vi "f_3_Qgtot_Vpl.vi"(0 "file path (IN)":path, 1 "Project #":string, 2 "Request #":string, 3 "TEST #":string, 5 "error in (no error)":errorcluster, 6 "VGE (-ve)":dbl, 8 "VGE (+ve)":dbl) -> (9 "Vpl":dbl, 11 "Di (A)":dbl, 13 "Dt (ns)":dbl, 14 "file path (OUT)":path, 15 "Qgtot - Delta Time (us)":dbl, 16 "Di/Dt (A/us)":dbl, 17 "DONE Qgtot & Vpl":bool, 18 "DONE Di/Dt ON":bool, 19 "error out":errorcluster)   [LabVIEW 2020]
uses:
  Global 1.vi
  <vilib>/measure/mamon.llb/Trigger Detection for 1 Channel.vi
  <vilib>/Analysis/NI_AALBase.lvlib
  <vilib>/measure/NI_MAPro.lvlib
panel:
  out "VGE (+ve) point":dbl
  out "Cursor c : Channel 2":dbl
  out "Find Major in Histogram":dbl
  out "Histogram":dynamicdata(graph)
  out "Focus graph":waveform(dbl)(graph)
  in  "Decision ?":bool
  out "Dt (us)":dbl
  out "VGE constant point in Median Filter":dbl
  out "VGE (-ve) point":dbl
  out "Cursor a : Channel 2":dbl
  out "Waveform Graph":waveform(dbl)[](graph)
  out "ON Region":waveform(dbl)[](graph) caption="Qgtot & Vpl"
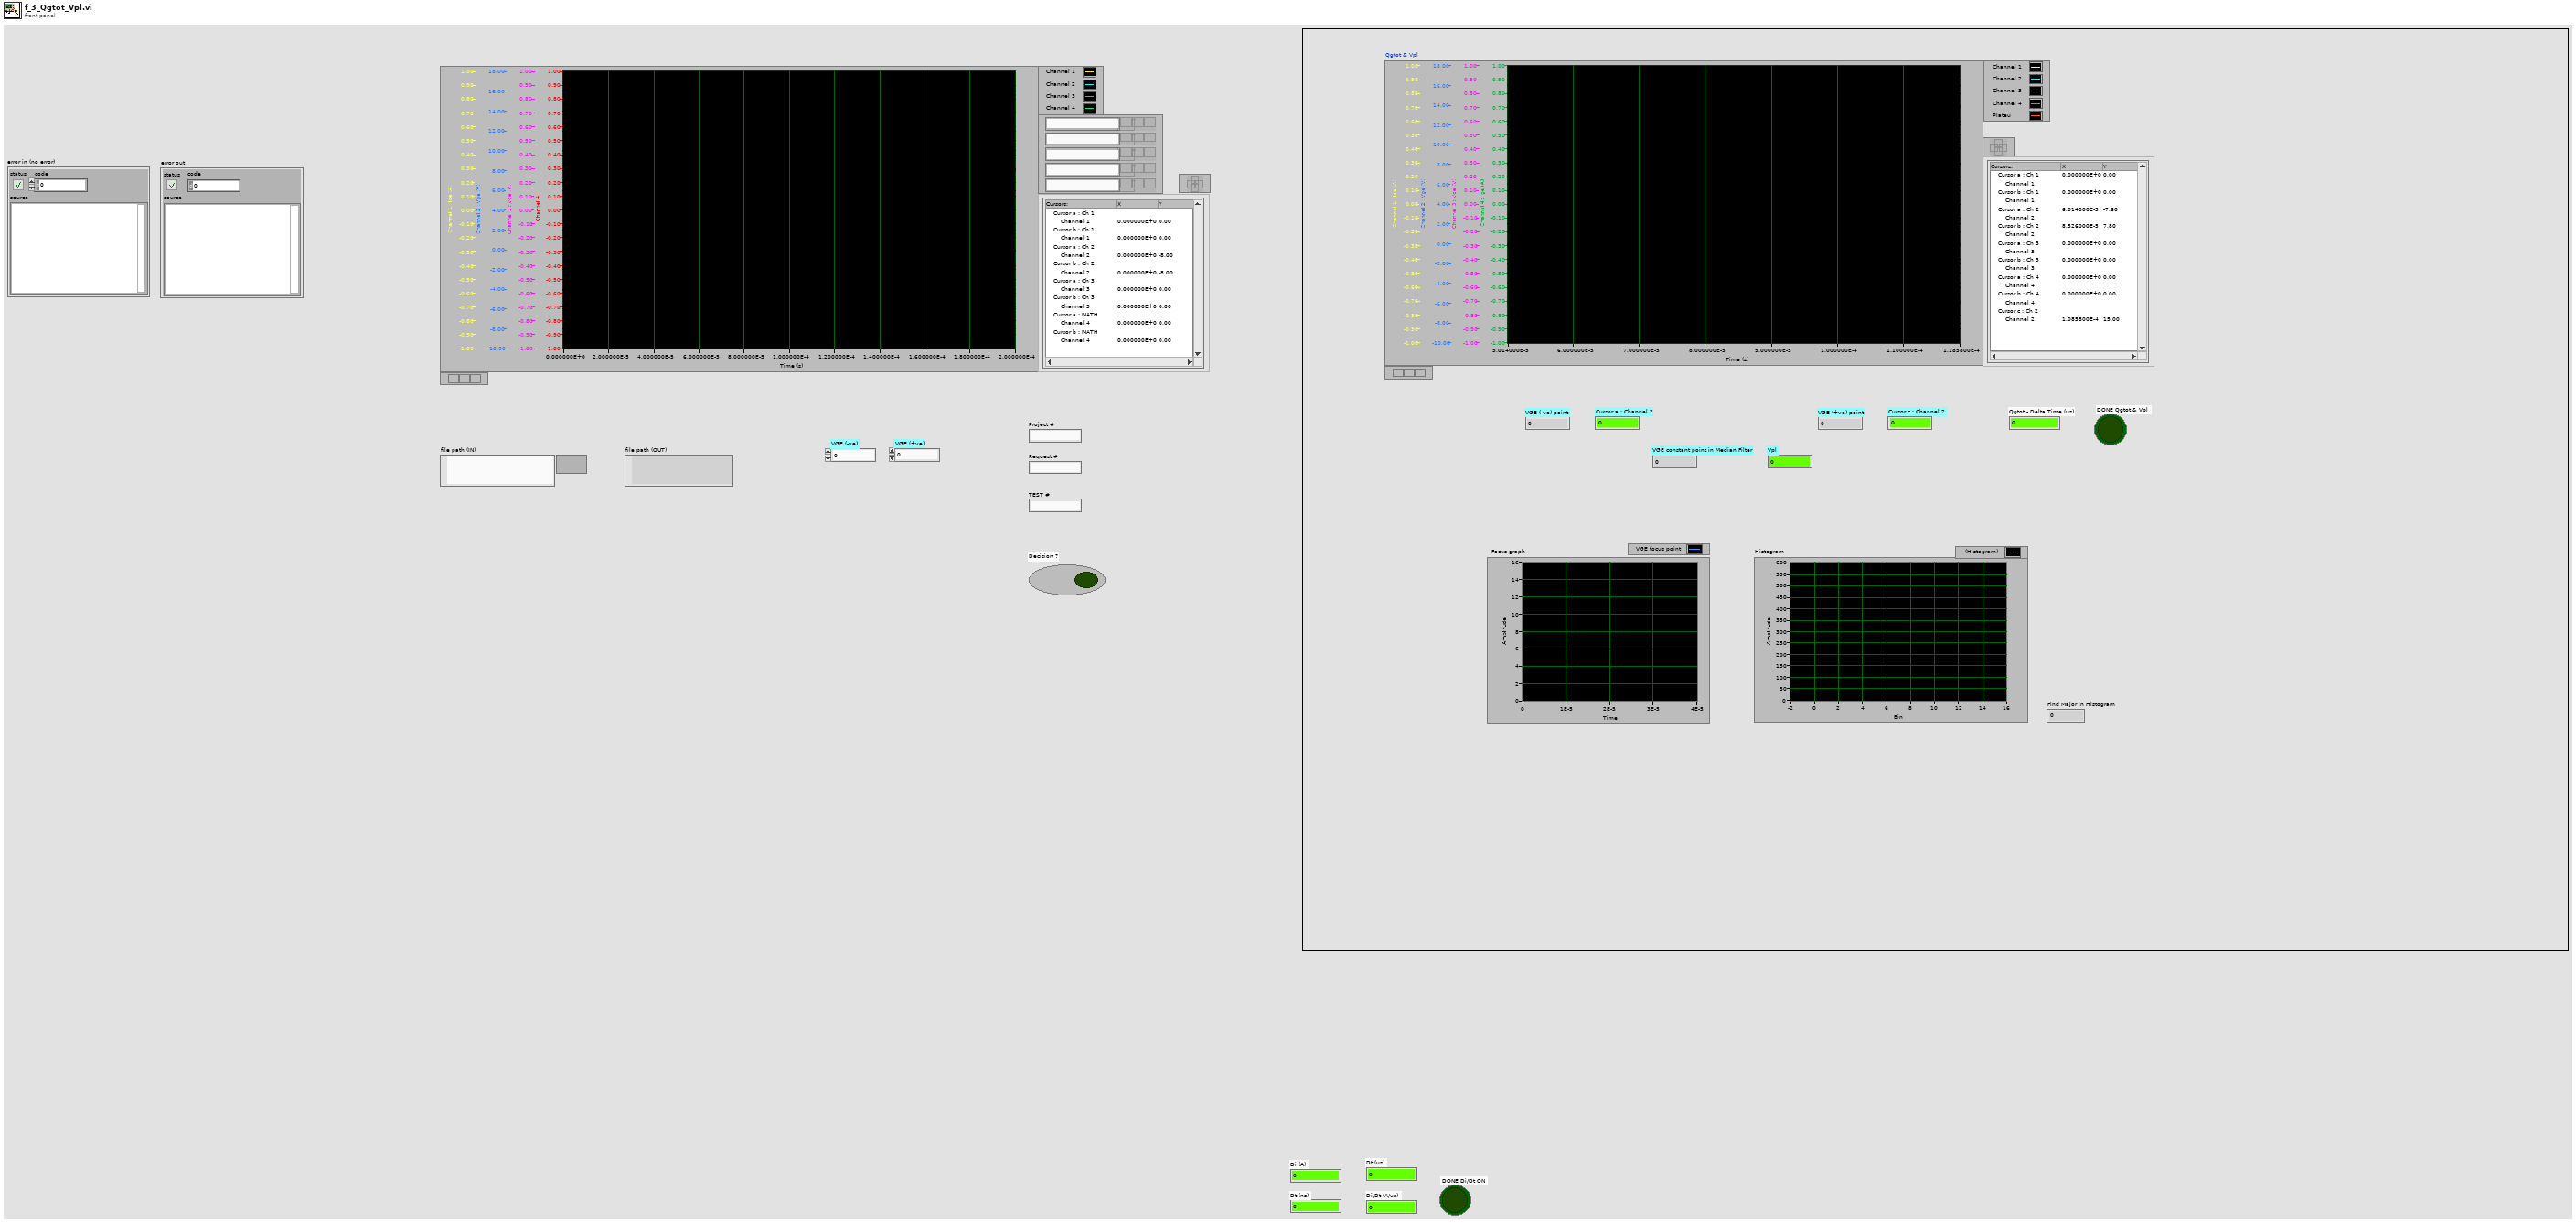
[diagram p1: front panel]
types:
  T1 = enum32{"Invalid", "Standard", "Closed", "Hidden", "Minimized", "Maximized"}
  T2 = typedef "imagedata.ctl" = cluster{"image type":i32, "image depth":i32, "image":u8[], "mask":u8[], "colors":u32[], "Rectangle":cluster{"left":i16, "top":i16, "right":i16, "bottom":i16}}
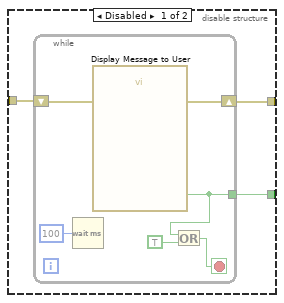
[diagram p2: hidden frame]
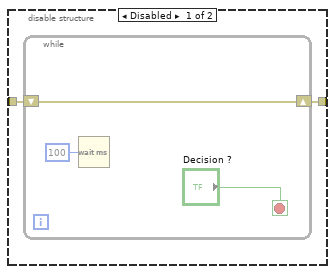
[diagram p10: hidden frame]
diagram:
  w5 = FALSE ("DONE Tdon")
  w1 = 0.0 ("Cursor a : Channel 1")
  w6 = errorcluster {"status"=FALSE, "code"=0, "source"=""} ("error out")
  w7 = waveform(dbl)[] [] ("Waveform Graph")
  n1 = local write "DONE Qgtot & Vpl"(w5) -> ()
  n2 = local write "VGE (-ve) point"(w1) -> ()
  n3 = local write "DONE Di/Dt ON"(w5) -> ()
  n4 = local write "Decision ?"(w5) -> ()
  n5 = local write "VGE constant point in Median Filter"(w1) -> ()
  n6 = local write "Di (A)"(w1) -> ()
  n7 = local write "Dt (ns)"(w1) -> ()
  n8 = local write "Dt (us)"(w1) -> ()
  n9 = local write "Di/Dt (A/us)"(w1) -> ()
  n10 = local write "VGE (+ve) point"(w1) -> ()
  n11 = local write "Cursor c : Channel 2"(w1) -> ()
  n12 = local write "Find Major in Histogram"(0.0 ("Time of Maximum")) -> ()
  n13 = local write "error out"(w6) -> ()
  n14 = local write "error in (no error)"(w6) -> ()
  n15 = local write "Cursor a : Channel 2"(w1) -> ()
  n16 = local write "Vpl"(w1) -> ()
  n17 = local write "Qgtot - Delta Time (us)"(w1) -> ()
  n18 = local write "Waveform Graph"(w7) -> ()
  n19 = local write "ON Region"(w7) -> ()
  n20 = local write "Histogram"(dynamicdata [] ("Histogram")) -> ()
  n21 = local write "Focus graph"(waveform(dbl) {"t0"=timestamp(0 s since 1904-01-01), "dt"=1.0, "Y"=[]} ("Focus graph")) -> ()
  n22 = flat-sequence {
    tunnel: ["file path (IN)"] -> w13
    tunnel: [w14] -> w12
    tunnel: [w23] -> w11
    tunnel: [w22] -> w10
    tunnel: w13 -> [w25]
    tunnel: w12 -> [w24]
    tunnel: [w314] -> w9
    tunnel: w11 -> [w313]
    tunnel: w10 -> [w312]
    tunnel: [w312] -> w8
    tunnel: w9 -> [w329]
    tunnel: w8 -> [w328]
    frame #0 {
      n23 = control-ref of="This VI"() -> (w19:refnum<vi>)
      n24 = invoke class="VI" method="FP.Open"(reference=w19, error in="error in (no error)", "Activate"=TRUE ("Activate?"), "State"=T1."Maximized") -> (error out=w20:errorcluster)  [unwired: 1 in, 4 out]
      n25 = property class="VI"(reference=w19, error in=w20, "Front Panel.Closeable"=TRUE ("Front Panel Window:Closeable")) -> (error out=w14:errorcluster)  [unwired: 1 out]
    }
    frame #1 {
      n26 = while {
        tunnel: w25 -> [w57]
        shift-right: [w52] -> w23
        shift-left: w24 -> [w56]
        tunnel: [w54] -> w22
        stop <- w51 stop-if-true
        n27 = flat-sequence {
          tunnel: [w86] -> w67
          tunnel: [w87] -> w66
          tunnel: w57 -> [w87]
          tunnel: w56 -> [w86]
          tunnel: w67 -> [w105]
          tunnel: w66 -> [w103]
          tunnel: [w102] -> w47
          tunnel: [w94] -> w46
          tunnel: [w88] -> w45
          tunnel: [w90] -> w44
          tunnel: [w91] -> w43
          tunnel: [w89] -> w42
          tunnel: [w92] -> w41
          tunnel: w47 -> [w145]
          tunnel: [w145] -> w40
          tunnel: w46 -> [w144]
          tunnel: [w144] -> w38
          tunnel: w45 -> [w136]
          tunnel: w44 -> [_]
          tunnel: w43 -> [w143]
          tunnel: w42 -> [w142]
          tunnel: [w142] -> w39
          tunnel: w41 -> [w141]
          tunnel: [w134] -> w37
          tunnel: [w157] -> w50
          tunnel: w40 -> [w215]
          tunnel: [w215] -> w49
          tunnel: w39 -> [w214]
          tunnel: [w214] -> w48
          tunnel: w38 -> [w171]
          tunnel: w37 -> [w164]
          tunnel: w50 -> [w228]
          tunnel: [w236] -> w36
          tunnel: w49 -> [w244]
          tunnel: [w244] -> w35
          tunnel: [w232] -> w33
          tunnel: [w229] -> w29
          tunnel: w48 -> [w216]
          tunnel: [w216] -> w26
          tunnel: w36 -> [w261]
          tunnel: w35 -> [w266]
          tunnel: [w266] -> w34
          tunnel: w33 -> [w265]
          tunnel: [w265] -> w32
          tunnel: [w249] -> w31
          tunnel: [w251] -> w30
          tunnel: w29 -> [w264]
          tunnel: [w264] -> w28
          tunnel: [w252] -> w27
          tunnel: w26 -> [w259]
          tunnel: [w269] -> w65
          tunnel: w34 -> [w274]
          tunnel: [w274] -> w64
          tunnel: w32 -> [w273]
          tunnel: [w273] -> w63
          tunnel: w31 -> [w272]
          tunnel: [w272] -> w62
          tunnel: w30 -> [w267]
          tunnel: [w267] -> w61
          tunnel: w28 -> [w271]
          tunnel: [w271] -> w60
          tunnel: w27 -> [w270]
          tunnel: w65 -> [w286]
          tunnel: w64 -> [w298]
          tunnel: [w298] -> w59
          tunnel: w63 -> [w293]
          tunnel: w62 -> [w294]
          tunnel: w61 -> [w292]
          tunnel: w60 -> [w291]
          tunnel: [w286] -> w58
          tunnel: w59 -> [w303]
          tunnel: w58 -> [w305]
          tunnel: [w304] -> w53
          tunnel: [w303] -> w54
          frame #0 {
            w83 = waveform(dbl)[] [] ("Waveform Graph")
            w79 = 0.0 ("Cursor a : Channel 1")
            w85 = FALSE ("DONE Tdon")
            n28 = local write "DONE Qgtot & Vpl"(w85) -> ()
            n29 = local write "Cursor a : Channel 2"(w79) -> ()
            n30 = local write "Di (A)"(w79) -> ()
            n31 = local write "Dt (ns)"(w79) -> ()
            n32 = local write "Dt (us)"(w79) -> ()
            n33 = local write "Di/Dt (A/us)"(w79) -> ()
            n34 = local write "DONE Di/Dt ON"(w85) -> ()
            n35 = local write "Decision ?"(w85) -> ()
            n36 = local write "Find Major in Histogram"(w79) -> ()
            n37 = local write "VGE constant point in Median Filter"(w79) -> ()
            n38 = local write "VGE (-ve) point"(w79) -> ()
            n39 = local write "VGE (+ve) point"(w79) -> ()
            n40 = local write "Cursor c : Channel 2"(w79) -> ()
            n41 = local write "Qgtot - Delta Time (us)"(w79) -> ()
            n42 = Wait (ms)(milliseconds to wait=u32 200) -> ()  [unwired: 1 out]
            n43 = local write "Vpl"(w79) -> ()
            n44 = Wait (ms)(milliseconds to wait=u32 200) -> ()  [unwired: 1 out]
            n45 = local write "Histogram"(dynamicdata [] ("Histogram")) -> ()
            n46 = local write "ON Region"(w83) -> ()
            n47 = local write "Waveform Graph"(w83) -> ()
            n48 = local write "Focus graph"(waveform(dbl) {"t0"=timestamp(0 s since 1904-01-01), "dt"=1.0, "Y"=[]} ("Focus graph")) -> ()
          }
          frame #1 {
            w94 = 0.0 ("number")
            # "Channel 2"
            # "Channel 4"
            # "t0"
            # "Channel 1"
            # "Channel 3"
            # "dt"
            # "Ch1"
            n49 = call "3_ReadDatatoWaveform.vi"("file path (IN)"=w103, "error in (no error)"=w105) -> ("Ch 1 Data"=w101:dbl[], "Ch 2 Data"=w96:dbl[], "file path (OUT)"=w102:path, "Waveform Graph"=→"Waveform Graph":waveform(dbl)[], "Ch 3 Data"=w100:dbl[], "Ch 4 Data"=w98:dbl[], "dt"=w91:dbl, "error out"=w104:errorcluster)  [unwired: 5 in, 1 out]
            n50 = To Time Stamp(1:w94) -> (0:w97:timestamp)
            n51 = disable-structure shown="Enabled" {
              disable-tunnel: w97 -> [w121 _]
              disable-tunnel: w91 -> [w120 _]
              disable-tunnel: w96 -> [w119 _]
              disable-tunnel: [w118 _] -> w90
              frame Enabled {
                # "Channel 2"
                n52 = Bundle By Name("Y"=w119, "dt"=w120, "t0"=w121) -> (w118:waveform(dbl))  [unwired: 1 in]
              }
              frame Disabled {
              }
            }
            n53 = disable-structure shown="Enabled" {
              disable-tunnel: w97 -> [w133 _]
              disable-tunnel: w91 -> [w132 _]
              disable-tunnel: w100 -> [w131 _]
              disable-tunnel: [w130 _] -> w106
              frame Enabled {
                # "Channel 3"
                n54 = Bundle By Name("Y"=w131, "dt"=w132, "t0"=w133) -> (w130:waveform(dbl))  [unwired: 1 in]
              }
              frame Disabled {
              }
            }
            n55 = disable-structure shown="Enabled" {
              disable-tunnel: w97 -> [w125 _]
              disable-tunnel: w91 -> [w124 _]
              disable-tunnel: w98 -> [w123 _]
              disable-tunnel: [w122 _] -> w93
              frame Enabled {
                # "Channel 4"
                n56 = Bundle By Name("Y"=w123, "dt"=w124, "t0"=w125) -> (w122:waveform(dbl))  [unwired: 1 in]
              }
              frame Disabled {
              }
            }
            n57 = disable-structure shown="Enabled" {
              disable-tunnel: w97 -> [w129 _]
              disable-tunnel: w91 -> [w128 _]
              disable-tunnel: w101 -> [w127 _]
              disable-tunnel: [w126 _] -> w107
              frame Enabled {
                # "Channel 1"
                n58 = Bundle By Name("Y"=w127, "dt"=w128, "t0"=w129) -> (w126:waveform(dbl))  [unwired: 1 in]
              }
              frame Disabled {
              }
            }
            n59 = property on="Waveform Graph" class="WFGraph (strict)"(error in=w104, "XScale.Offset"=w94) -> (error out=w88:errorcluster)  [unwired: 1 in, 1 out]
            n60 = disable-structure shown="Enabled" {
              disable-tunnel: w90 -> [w116 _]
              disable-tunnel: [w115 _] -> w89
              disable-tunnel: [w114 _] -> w92
              disable-tunnel: w91 -> [w113 _]
              frame Enabled {
                # "OG = 30"
                # "Median"
                n61 = global read "Global 1.vi" "Median Filter Rank"() -> (w112:i32)
                n62 = Unbundle By Name(w116) -> ("Y"=w117:dbl[])
                n63 = call <vilib>:"Median Filter.vi"("right rank"=w112, "left rank"=w112, "X"=w117) -> ("Filtered X"=w114:dbl[])  [unwired: 7 in, 1 out]
                n64 = Bundle By Name("Y"=w114, "dt"=w113) -> (w115:waveform(dbl))  [unwired: 1 in]
              }
              frame Disabled {
              }
            }
            n65 = Build Array(w107, w90, w106, w93, w89) -> (→"ON Region":waveform(dbl)[])
            n66 = Wait (ms)(milliseconds to wait=u32 200) -> ()  [unwired: 1 out]
            n67 = call <vilib>:"Beep.vi"("use system alert? (T)"=FALSE, "duration (msec)"=u32 200, "frequency (Hz)"=u32 2000) -> ()  [unwired: 9 in]
          }
          frame #2 {
            n68 = disable-structure shown="Enabled" {
              disable-tunnel: w143 -> [_ w151]
              disable-tunnel: w141 -> [_ w147]
              disable-tunnel: [_ w146] -> w139
              frame Disabled {
              }
              frame Enabled {
                # "Remains"
                # "Find (+ve)"
                # "Find 0"
                n69 = Search 1D Array(1D array=w147, element=0.0, start index (0)=0) -> (index of element=w152:i32)
                n70 = Split 1D Array(array=w147, index=w152) -> (second subarray=w155:dbl[])  [unwired: 1 out]
                n71 = Search 1D Array(1D array=w155, element="VGE (+ve)", start index (0)=0) -> (index of element=w154:i32)
                n72 = Split 1D Array(array=w155, index=w154) -> (first subarray=w156:dbl[])  [unwired: 1 out]
                n73 = Bundle By Name("Y"=w156, "dt"=w151) -> (w146:waveform(dbl))  [unwired: 1 in]
                "Focus graph" <- w146
              }
            }
            n74 = Wait (ms)(milliseconds to wait=u32 200) -> ()  [unwired: 1 out]
            n75 = call "Create Histogram"("error in (no error)"=w136, "Signal"=w139) -> ("error out"=w135:errorcluster, "Histogram"=w138:dynamicdata)  [unwired: 8 in]
            "Histogram" <- w138
            n76 = call "Statistics"("Signals"=w138, "error in (no error)"=w135) -> ("Time of Maximum"=→"Find Major in Histogram":dynamicdata, "error out"=w134:errorcluster)  [unwired: 24 in]
          }
          frame #3 {
            n77 = property on="ON Region" class="WFGraph (strict)"(error in=w164) -> (error out=w172:errorcluster, "Width"=w173:u32)  [unwired: 1 in, 1 out]
            n78 = property on="ON Region" class="WFGraph (strict)"(error in=w172, "Caption.Justify"=enum16{"Left", "Center", "Right"}."Left" ("Caption.Justification"), "Caption.Width"=w173, "Caption.FontBold"=TRUE ("Caption.Font:Bold"), "Caption.FontColor"=u32 16860 ("Caption.Font:Color"), "Caption.FontSize"=u32 24 ("Caption.Font:Size"), "Caption.Text"="Qgtot & Vpl") -> (error out=w174:errorcluster)  [unwired: 1 in, 1 out]
            n79 = Wait (ms)(milliseconds to wait=u32 200) -> ()  [unwired: 1 out]
            n80 = property on="ON Region" class="WFGraph (strict)"(error in=w174, "XScale.Offset"=w171) -> (error out=w165:errorcluster)  [unwired: 1 in, 1 out]
            n81 = property on="ON Region" class="WFGraph (strict)"(error in=w165, "Active Cursor"=u32 0, "Cursor.Cursor X"=0.0 ("Cursor.Cursor Position:Cursor X"), "Cursor.Cursor Y"=0.0 ("Cursor.Cursor Position:Cursor Y"), "Cursor.Visible"=FALSE) -> (error out=w207:errorcluster)  [unwired: 1 in, 1 out]
            n82 = property on="ON Region" class="WFGraph (strict)"(error in=w207, "Active Cursor"=u32 1, "Cursor.Cursor X"=0.0 ("Cursor.Cursor Position:Cursor X"), "Cursor.Cursor Y"=0.0 ("Cursor.Cursor Position:Cursor Y"), "Cursor.Visible"=FALSE) -> (error out=w208:errorcluster)  [unwired: 1 in, 1 out]
            n83 = property on="ON Region" class="WFGraph (strict)"(error in=w208, "Active Cursor"=u32 2, "Cursor.Cursor X"=0.0 ("Cursor.Cursor Position:Cursor X"), "Cursor.Cursor Y"=0.0 ("Cursor.Cursor Position:Cursor Y"), "Cursor.Visible"=FALSE) -> (error out=w209:errorcluster)  [unwired: 1 in, 1 out]
            n84 = property on="ON Region" class="WFGraph (strict)"(error in=w209, "Active Cursor"=u32 3, "Cursor.Cursor X"=0.0 ("Cursor.Cursor Position:Cursor X"), "Cursor.Cursor Y"=0.0 ("Cursor.Cursor Position:Cursor Y"), "Cursor.Visible"=FALSE) -> (error out=w210:errorcluster)  [unwired: 1 in, 1 out]
            n85 = property on="ON Region" class="WFGraph (strict)"(error in=w210, "Active Cursor"=u32 4, "Cursor.Cursor X"=0.0 ("Cursor.Cursor Position:Cursor X"), "Cursor.Cursor Y"=0.0 ("Cursor.Cursor Position:Cursor Y"), "Cursor.Visible"=FALSE) -> (error out=w211:errorcluster)  [unwired: 1 in, 1 out]
            n86 = property on="ON Region" class="WFGraph (strict)"(error in=w211, "Active Cursor"=u32 5, "Cursor.Cursor X"=0.0 ("Cursor.Cursor Position:Cursor X"), "Cursor.Cursor Y"=0.0 ("Cursor.Cursor Position:Cursor Y"), "Cursor.Visible"=FALSE) -> (error out=w212:errorcluster)  [unwired: 1 in, 1 out]
            n87 = property on="ON Region" class="WFGraph (strict)"(error in=w212, "Active Cursor"=u32 6, "Cursor.Cursor X"=0.0 ("Cursor.Cursor Position:Cursor X"), "Cursor.Cursor Y"=0.0 ("Cursor.Cursor Position:Cursor Y"), "Cursor.Visible"=FALSE) -> (error out=w213:errorcluster)  [unwired: 1 in, 1 out]
            n88 = property on="ON Region" class="WFGraph (strict)"(error in=w213, "Active Cursor"=u32 7, "Cursor.Cursor X"=0.0 ("Cursor.Cursor Position:Cursor X"), "Cursor.Cursor Y"=0.0 ("Cursor.Cursor Position:Cursor Y"), "Cursor.Visible"=FALSE) -> (error out=w158:errorcluster)  [unwired: 1 in, 1 out]
            n89 = property on="ON Region" class="WFGraph (strict)"(error in=w158, "Active Cursor"=u32 8, "Cursor.Cursor X"=0.0 ("Cursor.Cursor Position:Cursor X"), "Cursor.Cursor Y"=0.0 ("Cursor.Cursor Position:Cursor Y"), "Cursor.Visible"=FALSE) -> (error out=w157:errorcluster)  [unwired: 1 in, 1 out]
          }
          frame #4 {
            w225 = u16 1 items=["Falling Edge", "Rising Edge"] ("trigger slope")
            w226 = u16 1 items=["Index", "Time"] ("location mode")
            w230 = u16 1 items=["Falling Edge", "Rising Edge"] ("trigger slope")
            w231 = u16 1 items=["Index", "Time"] ("location mode")
            # "Cursor a : Channel 2"
            # "Cursor a : Channel 2"
            # "Cursor b : Channel 2"
            # "Cursor a : Channel 2"
            # "Cursor b : Channel 2"
            # "Cursor a : Channel 2"
            # "End Time 1st Cursor"
            # "End Time 2nd Cursor"
            # "1st PARAMETER : VGE (-ve)"
            # "Channel 2"
            # "2nd PARAMETER : VGE constant point"
            # "Channel 2"
            n90 = Add(x="VGE (-ve)", y=0.3) -> (x+y=w219:dbl)
            n91 = call-poly <vilib>:"Basic Level Trigger Detection.vi"("signal in"=w216, "level"=w219, "location mode"=w231, "error in (no error)"=w228, "trigger slope"=w230) -> ("trigger location"=w229:dbl, "error out"=w227:errorcluster)  [unwired: 8 in, 1 out]
            n92 = property on="ON Region" class="WFGraph (strict)"(error in=w227, "Active Cursor"=u32 2, "Cursor.Cursor X"=w229, "Cursor.Visible"=TRUE, "Cursor.Cursor Name Visible"=TRUE) -> (error out=w240:errorcluster)  [unwired: 1 in, 1 out]
            n93 = property on="ON Region" class="WFGraph (strict)"(error in=w240, "Active Cursor"=u32 2) -> (error out=w222:errorcluster, "Cursor.Cursor Y"=w232:dbl)  [unwired: 1 in, 1 out]
            "Cursor a : Channel 2" <- w232
            n94 = local read "Find Major in Histogram"() -> (w221:dbl)
            "VGE constant point in Median Filter" <- w221
            n95 = call-poly <vilib>:"Basic Level Trigger Detection.vi"("signal in"=w216, "level"=w221, "location mode"=w226, "error in (no error)"=w222, "trigger slope"=w225) -> ("trigger location"=w223:dbl, "error out"=w224:errorcluster)  [unwired: 8 in, 1 out]
            n96 = Wait (ms)(milliseconds to wait=u32 200) -> ()  [unwired: 1 out]
            n97 = property on="ON Region" class="WFGraph (strict)"(error in=w224, "Active Cursor"=u32 3, "Cursor.Cursor X"=w223, "Cursor.Visible"=TRUE, "Cursor.Cursor Name Visible"=TRUE) -> (error out=w237:errorcluster)  [unwired: 1 in, 1 out]
            n98 = call <vilib>:"Beep.vi"("use system alert? (T)"=FALSE, "duration (msec)"=u32 200, "frequency (Hz)"=u32 2000) -> ()  [unwired: 9 in]
            n99 = property on="ON Region" class="WFGraph (strict)"(error in=w237, "Active Cursor"=u32 3) -> (error out=w236:errorcluster, "Cursor.Cursor Y"=→"Vpl":dbl)  [unwired: 1 in, 1 out]
            "VGE (-ve) point" <- "VGE (-ve)"
          }
          frame #5 {
            w263 = u16 1 items=["Falling Edge", "Rising Edge"] ("trigger slope")
            w262 = u16 1 items=["Index", "Time"] ("location mode")
            # "Cursor c : Channel 2"
            # "Cursor c : Channel 2"
            # "VGE +ve"
            # "Channel 2"
            n100 = local read "VGE (+ve)"() -> (w250:dbl)
            "VGE (+ve) point" <- w250
            n101 = call-poly <vilib>:"Basic Level Trigger Detection.vi"("signal in"=w259, "level"=w250, "location mode"=w262, "error in (no error)"=w261, "trigger slope"=w263) -> ("trigger location"=w251:dbl, "error out"=w253:errorcluster)  [unwired: 8 in, 1 out]
            n102 = property on="ON Region" class="WFGraph (strict)"(error in=w253, "Active Cursor"=u32 8, "Cursor.Cursor X"=w251, "Cursor.Visible"=TRUE, "Cursor.Cursor Name Visible"=TRUE) -> (error out=w257:errorcluster)  [unwired: 1 in, 1 out]
            n103 = property on="ON Region" class="WFGraph (strict)"(error in=w257, "Active Cursor"=u32 8) -> (error out=w252:errorcluster, "Cursor.Cursor Y"=w249:dbl)  [unwired: 1 in, 1 out]
            "Cursor c : Channel 2" <- w249
            n104 = Wait (ms)(milliseconds to wait=u32 200) -> ()  [unwired: 1 out]
          }
          frame #6 {
            n105 = disable-structure shown="Enabled" {
              disable-tunnel: w270 -> [w282 w283]
              disable-tunnel: [w281 w283] -> w269
              disable-tunnel: w271 -> [w276 _]
              disable-tunnel: w267 -> [w275 _]
              frame Enabled {
                # "2nd Cursor"
                # "1st Cursor"
                n106 = Subtract(x=w276, y=1e-05) -> (x-y=w277:dbl)
                n107 = Add(x=w275, y=1e-05) -> (x+y=w278:dbl)
                n108 = property on="ON Region" class="WFGraph (strict)"(error in=w282, "XScale.Minimum"=w277, "XScale.Maximum"=w278) -> (error out=w281:errorcluster)  [unwired: 1 in, 1 out]
              }
              frame Disabled {
              }
            }
            n109 = Wait (ms)(milliseconds to wait=u32 200) -> ()  [unwired: 1 out]
          }
          frame #7 {
            # "us"
            # "ns"
            n110 = Subtract(x=w294, y=w293) -> (x-y=w289:dbl)
            n111 = Subtract(x=w292, y=w291) -> (x-y=w290:dbl)
            n112 = Absolute Value(x=w289) -> (abs(x)=w288:dbl)
            "Di (A)" <- w288
            n113 = Absolute Value(x=w290) -> (abs(x)=w287:dbl)
            n114 = Multiply(x=w287, y=1000000.0) -> (x*y=w284:dbl)
            "Dt (us)" <- w284
            "Qgtot - Delta Time (us)" <- w284
            n115 = Multiply(x=w287, y=1000000000.0) -> (x*y=→"Dt (ns)":dbl)
            n116 = call <vilib>:"Beep.vi"("use system alert? (T)"=FALSE, "duration (msec)"=u32 200, "frequency (Hz)"=u32 2000) -> ()  [unwired: 9 in]
            n117 = Wait (ms)(milliseconds to wait=u32 200) -> ()  [unwired: 1 out]
            n118 = Divide(x=w288, y=w284) -> (x/y=→"Di/Dt (A/us)":dbl)
          }
          frame #8 {
            n119 = disable-structure shown="Enabled" {
              disable-tunnel: w305 -> [w307 w311]
              disable-tunnel: [w306 w311] -> w304
              frame Disabled {
                n120 = while {
                  shift-right: [w308] -> w306
                  shift-left: w307 -> [w308]
                  stop <- "Decision ?" stop-if-true
                  n121 = Wait (ms)(milliseconds to wait=u32 100) -> ()  [unwired: 1 out]
                }
              }
              frame Enabled {
              }
            }
          }
        }
        n122 = disable-structure shown="Enabled" {
          disable-tunnel: w53 -> [w70 w77]
          disable-tunnel: [w69 w77] -> w52
          disable-tunnel: [w68 TRUE ("NO")] -> w51
          frame Disabled {
            n123 = while {
              tunnel: [w72] -> w68
              shift-right: [w75] -> w69
              shift-left: w70 -> [w76]
              stop <- w74 stop-if-true
              n124 = Wait (ms)(milliseconds to wait=u32 100) -> ()  [unwired: 1 out]
              n125 = call "Display Message to User"("error in (no error)"=w76) -> ("error out"=w75:errorcluster, "NO"=w72:bool)  [unwired: 9 in]
              n126 = Or(x=w72, y=TRUE) -> (x .or. y?=w74:bool)
            }
          }
          frame Enabled {
          }
        }
        n127 = Wait (ms)(milliseconds to wait=u32 100) -> ()  [unwired: 1 out]
      }
    }
    frame #2 {
      w317 = "_"
      n128 = invoke on="ON Region" class="WFGraph (strict)" method="Get Image"(error in=w313) -> (error out=w321:errorcluster, "image data"=w324:T2)  [unwired: 5 in, 4 out]
      n129 = Concatenate Strings("C:\\GateCharge_Project\\GateCharge_Image\\" ("string"), "Project #", w317, "Request #", w317, "TEST #", w317, "Qgtot_Vpl" ("string"), ".png" ("string")) -> (w325:string)
      n130 = String To Path(string=w325) -> (path=w323:path)
      n131 = call <vilib>:"Write PNG File.vi"("error in (no error)"=w321, "image data"=w324, "path to PNG file"=w323) -> ("error out"=w314:errorcluster)  [unwired: 7 in, 1 out]
      "DONE Qgtot & Vpl" <- TRUE ("DONE Tdon")
      "DONE Di/Dt ON" <- TRUE ("DONE Di/Dt ON")
    }
    frame #3 {
      n132 = disable-structure shown="Enabled" {
        disable-tunnel: w329 -> [w330 _]
        frame Enabled {
          n133 = control-ref of="This VI"() -> (w331:refnum<vi>)
          n134 = invoke class="VI" method="FP.Close"(reference=w331, error in=w330) -> ()  [unwired: 1 in, 3 out]
        }
        frame Disabled {
        }
      }
      "error out" <- w329
      "file path (OUT)" <- w328
    }
  }
